vi "SMU_Only4Wire Resistance Configure SMU.vi"(7 "SMU Settings":T2={"Level"=0.01, "Level Range"=0.1, "Limit"=1.0, "Limit Range"=6.0, "Sense"=0} {"Sense" items=["Local"=1008, "Remote"=1009]}, 8 "error in (no error)":errorcluster, 9 "Published Data Id":string, 10 "Pins":string[](array[string]), 11 "Semiconductor Module Context":T3) -> (0 "error Out":errorcluster, 2 "R Array":dbl[](array[numeric]), 3 "Semiconductor Module Context Out":T3)   [LabVIEW 2013]
uses:
  <vilib>/NI_TestStand_SemiconductorModule/NI_TestStand_Semiconductor_Module.lvlibp/PinMap/General/SemiconductorModuleContext.ctl
  <instrlib>/niDCPower/nidcpower.llb/niDCPower Sense.ctl
  <vilib>/NI_TestStand_SemiconductorModule/NI_TestStand_Semiconductor_Module.lvlibp/PinMap/DC Power/PinsToNIDCPowerSessions.vi
  <vilib>/NI_TestStand_SemiconductorModule/NI_TestStand_Semiconductor_Module.lvlibp/PinMap/General/Publish/PublishDataDoubleFunctionalTest.vi
  <vilib>/NI_TestStand_SemiconductorModule/NI_TestStand_Semiconductor_Module.lvlibp
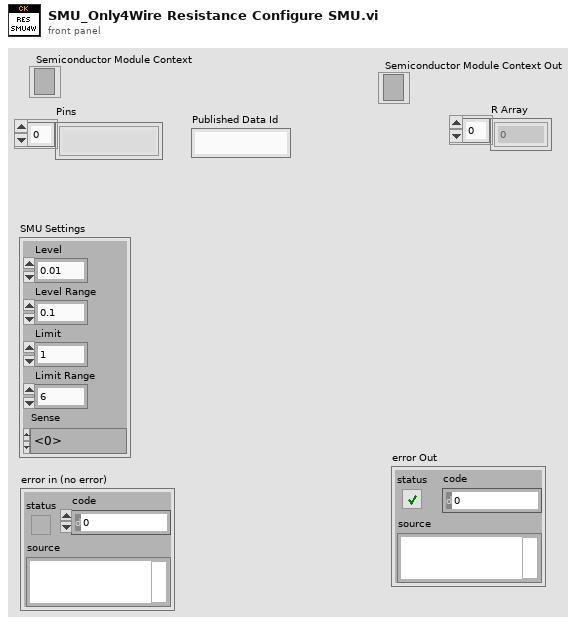
[diagram p1: front panel]
types:
  T1 = typedef "niDCPower Sense.ctl" = i32
  T2 = cluster{"Level":dbl, "Level Range":dbl, "Limit":dbl, "Limit Range":dbl, "Sense":T1}
  T3 = typedef "NI_TestStand_Semiconductor_Module.lvlibp/SemiconductorModuleContext.ctl" = refnum<k7>
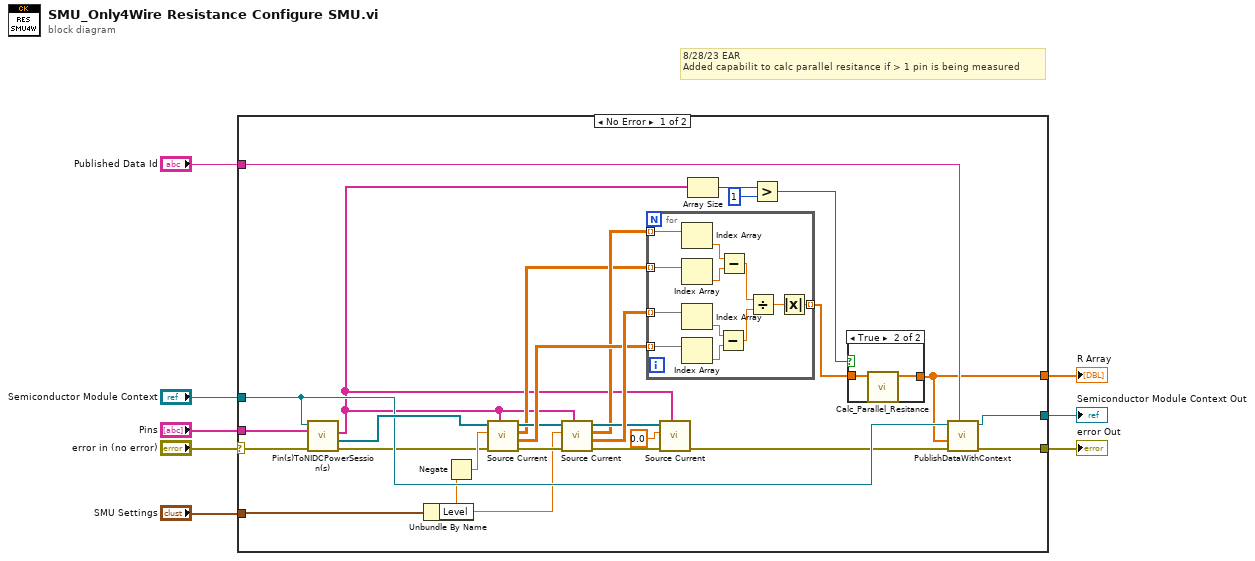
[diagram p0: block diagram]
diagram:
  # "8/28/23 EAR\nAdded capabilit to calc parallel resitance if > 1 pin is being measured"
  n1 = case shown="No Error" "error in (no error)" {
    selector: "error in (no error)" -> [w34 w52]
    tunnel: "Semiconductor Module Context" -> [w22 w51]
    tunnel: "Pins" -> [w23 _]
    tunnel: [w17 w52] -> w5
    tunnel: "Published Data Id" -> [w35 _]
    tunnel: [w28 w51] -> w3
    tunnel: [w10 _] -> w2
    tunnel: "SMU Settings" -> [w21 _]
    frame No Error {
      n2 = call-poly <vilib>:"Pin(s)ToNIDCPowerSession(s).vi"("error in (no error)"=w34, "Pins"=w23, "Semiconductor Module Context"=w22) -> ("error out"=w16:errorcluster, "Instrument Sessions"=w31:refnum<k15>[], "Channel Lists"=w14:string[])  [unwired: 4 in, 2 out]
      n3 = Unbundle By Name(w21) -> ("Level"=w20:dbl)
      n4 = Negate(x=w20) -> (-x=w29:dbl)
      n5 = call "Source Current.vi"("Channel Lists"=w14, "error in (no error)"=w16, "current level"=w29, "Instrument Sessions In"=w31) -> ("error out"=w26:errorcluster, "current measurements"=w32:dbl[][], "voltage measurements"=w24:dbl[][], "Instrument Sessions Out"=w25:refnum<k15>[])  [unwired: 4 in]
      n6 = call "Source Current.vi"("Channel Lists"=w14, "error in (no error)"=w26, "current level"=w20, "Instrument Sessions In"=w25) -> ("error out"=w19:errorcluster, "current measurements"=w33:dbl[][], "voltage measurements"=w27:dbl[][], "Instrument Sessions Out"=w30:refnum<k15>[])  [unwired: 4 in]
      n7 = for {
        tunnel: w27 -> [w42] mode=indexing
        tunnel: w33 -> [w50] mode=indexing
        tunnel: [w48] -> w11 mode=indexing
        tunnel: w32 -> [w46] mode=indexing
        tunnel: w24 -> [w39] mode=indexing
        n8 = Index Array(array=w42) -> (element=w41:dbl)  [unwired: 1 in]
        n9 = Index Array(array=w39) -> (element=w40:dbl)  [unwired: 1 in]
        n10 = Index Array(array=w50) -> (element=w43:dbl)  [unwired: 1 in]
        n11 = Index Array(array=w46) -> (element=w45:dbl)  [unwired: 1 in]
        n12 = Subtract(x=w43, y=w45) -> (x-y=w44:dbl)
        n13 = Subtract(x=w41, y=w40) -> (x-y=w47:dbl)
        n14 = Divide(x=w47, y=w44) -> (x/y=w49:dbl)
        n15 = Absolute Value(x=w49) -> (abs(x)=w48:dbl)
      }
      n16 = call "Source Current.vi"("Channel Lists"=w14, "error in (no error)"=w19, "current level"=0.0, "Instrument Sessions In"=w30) -> ("error out"=w18:errorcluster)  [unwired: 4 in, 3 out]
      n17 = Array Size(array=w14) -> (size(s)=w13:i32)
      n18 = Greater?(x=w13, y=1) -> (0:w9:bool)
      n19 = case shown="True" w9 {
        tunnel: w11 -> [w36 w38]
        tunnel: [w36 w37] -> w10
        frame False {
        }
        frame True {
          n20 = call "Calc_Parallel_Resitance.vi"("Resitance_Per Site"=w38) -> ("Parralel_Resistance"=w37:dbl[])  [unwired: 10 in]
        }
      }
      n21 = call-poly <vilib>:"PublishDataWithContext.vi"("Published Data Id"=w35, "error in (no error)"=w18, "Data In"=w10, "Semiconductor Module Context"=w22) -> ("error out"=w17:errorcluster, "Semiconductor Module Context Out"=w28:T3)  [unwired: 6 in]
    }
    frame Error {
    }
  }
  "error Out" <- w5
  "Semiconductor Module Context Out" <- w3
  "R Array" <- w2
